vi "Disabled.vi"(7 "Robot Mode":T2=enum."Teleop Disabled", 10 "Match Info":T1={"Autonomous Elapsed Seconds"=0.0, "TeleOp Elapsed Seconds"=0.0, "Disabled Elapsed Seconds"=93.761, "Visited Autonomous"=FALSE, "Visited TeleOp"=FALSE, "Visited Disabled"=TRUE, "Autonomous Settings"={"Autonomous Style"=enum."Independent", "VI Refnum"=refnum}}, 11 "Call Context":T3=enum."Execute") -> ()   [LabVIEW 2013]
doc: "This VI is called each time a disabled packet is received from the DS. It is often used to prepare for the next robot mode, to calibrate sensors, etc."
uses:
  <vilib>/Rock Robotics/WPI/DriverStation/WPI_DriverStationDerivedRobotMode.ctl
  <vilib>/Rock Robotics/WPI/DriverStation/WPI_DriverStationRobotMode2.ctl
  <vilib>/Rock Robotics/WPI/DriverStation/WPI_DriverStationMatch Info.ctl
  SonarAction.ctl
  Example_Code/PressureSensor/PressureSensorAction.ctl
  SingleSolenoidAction.ctl
  RefnameEnum.ctl
  TankDriveAction.ctl
panel:
  in  "AutoID":i32=3061
  out "LCDTimer":u32=121
  out "LCDIterations":i32
  out "error out":errorcluster
  in  "error in":errorcluster
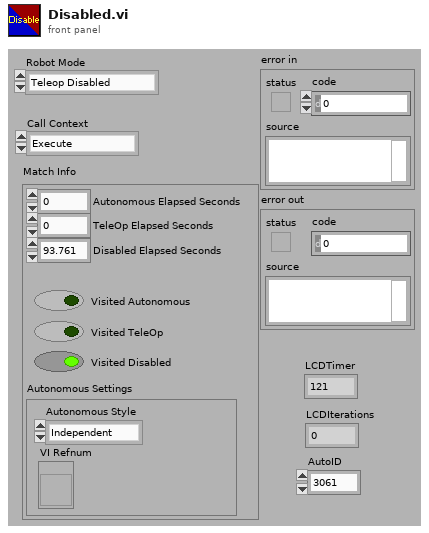
[diagram p1: front panel]
types:
  T1 = typedef "WPI_DriverStationMatch Info.ctl" = cluster{"Autonomous Elapsed Seconds":dbl, "TeleOp Elapsed Seconds":dbl, "Disabled Elapsed Seconds":dbl, "Visited Autonomous":bool, "Visited TeleOp":bool, "Visited Disabled":bool, "Autonomous Settings":cluster{"Autonomous Style":enum16{"Iterative", "Independent"}, "VI Refnum":refnum<vi>}}
  T2 = typedef "WPI_DriverStationRobotMode2.ctl" = enum16{"Autonomous Disabled", "Autonomous Enabled", "Teleop Disabled", "Teleop Enabled", "Timeout", "Finish", "Test Disabled", "Test Enabled"}
  T3 = typedef "WPI_DriverStationDerivedRobotMode.ctl" = enum16{"Init", "Execute", "Stop"}
  T4 = typedef "TankDriveAction.ctl" = enum16{"Init", "LinearDrive", "SetValue", "Disable"}
  T5 = typedef "RefnameEnum.ctl" = enum16{"TankDrive", "Controller1", "Controller2", "SonicShifter", "Compressor"}
  T6 = typedef "SingleSolenoidAction.ctl" = enum16{"Init", "SetState", "Disable"}
  T7 = typedef "WPI_SolenoidDevRef.ctl" = cluster{"DevStatus":errorcluster, "Solenoid Module":T8, "Forward Solenoid Channel":T9, "Reverse Solenoid Channel":T9}
  T8 = typedef "FPGA_TypedefSolenoidModule.ctl" = enum16{"Solenoid Module 1", "Solenoid Module 2"}
  T9 = typedef "WPI_SolenoidChannel.ctl" = enum8{"Solenoid 1", "Solenoid 2", "Solenoid 3", "Solenoid 4", "Solenoid 5", "Solenoid 6", "Solenoid 7", "Solenoid 8", "Invalid"}
  T10 = typedef "PressureSensorAction.ctl" = enum16{"Init", "ReadValue", "Disable"}
  T11 = typedef "SonarAction.ctl" = enum16{"Init", "ReadValue", "Disable"}
  T12 = typedef "AutoMode.ctl" = enum16{"OneBallFront", "OneBallCollector", "TwoBallNormal", "TwoBallHot"}
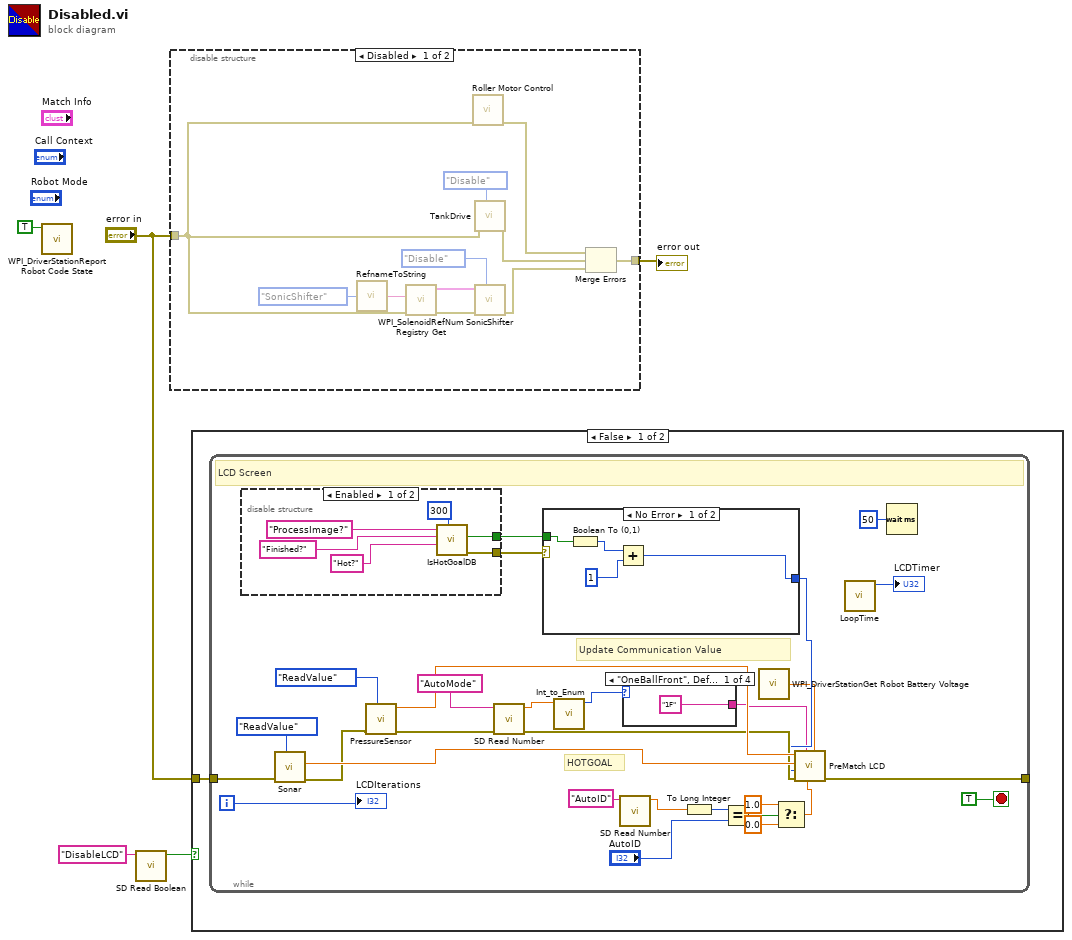
[diagram p0: block diagram]
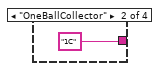
[diagram p3: hidden frame]
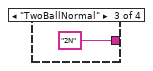
[diagram p4: hidden frame]
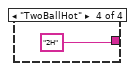
[diagram p5: hidden frame]
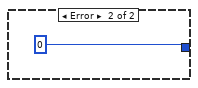
[diagram p6: hidden frame]
diagram:
  n1 = call <vilib>:"WPI_DriverStationReport Robot Code State.vi"("Disabled"=TRUE ("Autonomous")) -> ()  [unwired: 10 in, 1 out]
  n2 = call <vilib>:"SD Read Boolean.vi"("Name"="DisableLCD") -> ("Boolean"=w2:bool)  [unwired: 8 in, 2 out]
  n3 = disable-structure shown="Disabled" {
    disable-tunnel: [w9 _] -> w4
    disable-tunnel: "error in" -> [w8 _]
    frame Disabled {
      n4 = call "RefnameToString.vi"("Enum"=RefnameEnum."SonicShifter") -> ("Refname"=w14:string)
      n5 = call <vilib>:"WPI_SolenoidRefNum Registry Get.vi"("error in (no error)"=w8, "refnum name"=w14) -> ("error out"=w12:errorcluster, "SolenoidDevRef"=w16:T7)  [unwired: 8 in]
      n6 = call "Roller Motor Control.vi"("Error in"=w8) -> ("Error out"=w7:errorcluster)  [unwired: 10 in]
      n7 = call "TankDrive.vi"("DriveAction"=TankDriveAction."Disable", "error in (no error)"=w8) -> ("error out"=w11:errorcluster)  [unwired: 8 in, 1 out]
      n8 = call "SonicShifter.vi"("Action"=SingleSolenoidAction."Disable" ("Mode"), "error in (no error)"=w12, "SolenoidDevRef"=w16) -> ("error out"=w10:errorcluster)  [unwired: 8 in]
      n9 = Merge Errors(w7, w11, w10) -> (w9:errorcluster)
    }
    frame Enabled {
    }
  }
  "error out" <- w4
  n10 = case shown="False" w2 {
    tunnel: "error in" -> [w17 _]
    frame False {
      n11 = while {
        tunnel: w17 -> [w44]
        tunnel: [w45] -> _
        i -> [w26]
        stop <- TRUE stop-if-true
        # "HOTGOAL"
        # "Update Communication Value"
        # "LCD Screen"
        n12 = disable-structure shown="Enabled" {
          disable-tunnel: [w52 _] -> w35
          disable-tunnel: [w51 _] -> w34
          frame Enabled {
            n13 = call "IsHotGoalDB.vi"("Timeout (ms)"=u32 300, "DBHot?"="Hot?", "DBFinished?"="Finished?", "DBStart"="ProcessImage?") -> ("error out"=w52:errorcluster, "Hot?"=w51:bool)  [unwired: 5 in, 1 out]
          }
          frame Disabled {
          }
        }
        n14 = call "Sonar.vi"("Action"=SonarAction."ReadValue", "error in (no error)"=w44) -> ("error out"=w41:errorcluster, "distance"=w43:dbl)  [unwired: 8 in]
        n15 = call "PressureSensor.vi"("Action"=PressureSensorAction."ReadValue", "error in (no error)"=w41) -> ("error out"=w38:errorcluster, "Pressure"=w40:dbl)  [unwired: 8 in]
        n16 = call <vilib>:"SD Read Number.vi"("error in"=w38, "Name"="AutoMode") -> ("error out"=w37:errorcluster, "Numeric"=w31:dbl)  [unwired: 7 in, 1 out]
        n17 = case shown="No Error" w35 {
          tunnel: w34 -> [w60 _]
          tunnel: [w57 0] -> w33
          frame No Error {
            n18 = Boolean To (0,1)(Boolean=w60) -> (0, 1=w59:i16)
            n19 = Add(x=w59, y=1) -> (x+y=w57:i32)
          }
          frame Error {
          }
        }
        n20 = call "Int_to_Enum.vi"("IntIn"=w31) -> ("EnumOut"=w30:T12)  [unwired: 10 in]
        n21 = call <vilib>:"SD Read Number.vi"("Name"="AutoID") -> ("Numeric"=w24:dbl)  [unwired: 8 in, 2 out]
        n22 = case shown="\"OneBallFront\", Default" w30 {
          tunnel: ["1F" "1C" "2N" "2H"] -> w29
          frame "OneBallFront", Default {
          }
          frame "OneBallCollector" {
          }
          frame "TwoBallNormal" {
          }
          frame "TwoBallHot" {
          }
        }
        n23 = To Long Integer(number=w24) -> (32bit integer=w23:i32)
        n24 = Equal?(x=w23, y="AutoID") -> (x = y?=w21:bool)
        n25 = call <vilib>:"WPI_DriverStationGet Robot Battery Voltage.vi"() -> ("robot battery voltage"=w32:dbl)  [unwired: 14 in, 1 out]
        n26 = Select(t=1.0, s=w21, f=0.0) -> (s? t:f=w18:dbl)
        n27 = call "PreMatch LCD.vi"("Battery Voltage"=w32, "Communication Value:"=w18, "Autonomous Mode"=w29, "error in"=w37, "Camera"=w33, "Distance"=w43, "PSI"=w40) -> ("error out"=w45:errorcluster)  [unwired: 4 in]
        n28 = call "LoopTime.vi"() -> ("LoopTime"=→"LCDTimer":u32)  [unwired: 11 in]
        n29 = Wait (ms)(milliseconds to wait=u32 50) -> ()  [unwired: 1 out]
        "LCDIterations" <- w26
      }
    }
    frame True {
    }
  }
